vi "Test Prepare Path Returns Default if Empty.vi"(11 "Test Case In":refnum<class "Report Plugin Test.lvclass">) -> (0 "error out":errorcluster, 3 "Test Case Out":refnum<class "Report Plugin Test.lvclass">)   [LabVIEW 2020, in "Report Plugin Test.lvclass"]
uses:
  Report Plugin Test.lvclass
  C:/git/astemes-lunit/source/Framework/Report Plugin/Report Plugin.lvclass
  C:/Program Files (x86)/National Instruments/LabVIEW 2020/vi.lib/Astemes/LUnit/Test Case.lvclass
  <vilib>/Astemes/LUnit/Test Case.lvclass/Test Case.ctl
  <vilib>/Astemes/LUnit/Core/LUnit Test Case/Private/Append Fail Result.vi
  <vilib>/Astemes/LUnit/Core/LUnit Test Case/Private/Append Pass Result.vi
  <vilib>/Astemes/LUnit/Core/LUnit Test Case/Private/Run In UI.vi
  <vilib>/Utility/error.llb/Clear Errors.vi
  source/Framework/Report Plugin/Report Plugin.lvclass
  <vilib>/Astemes/LUnit/Test Case.lvclass
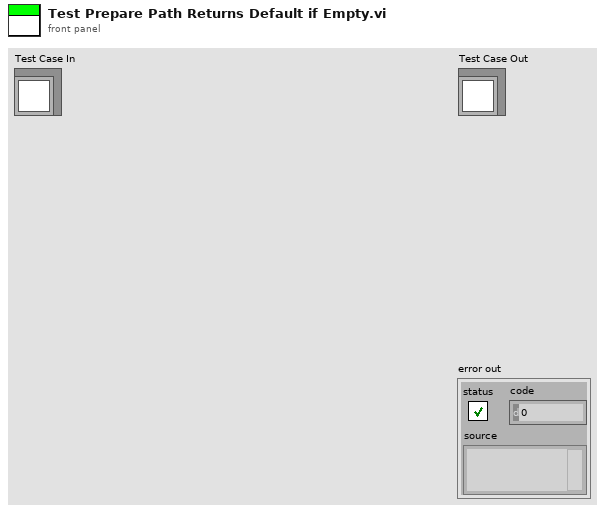
[diagram p1: front panel]
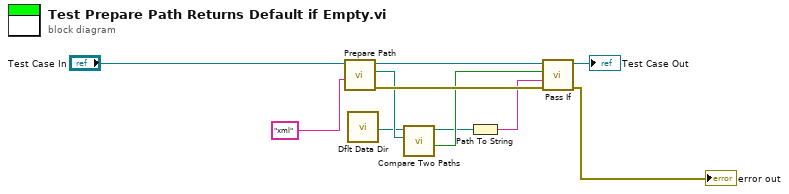
[diagram p0: block diagram]
diagram:
  n1 = call "Prepare Path.vi"("Extenssion"="xml", "Plugin In"="Test Case In") -> ("error out"=w7:errorcluster, "Modified Path"=w5:path, "Plugin Out"=w8:refnum<class "Report Plugin Test.lvclass">)  [unwired: 7 in]
  n2 = call <vilib>:"Dflt Data Dir.vi"() -> ("App:Default Data Directory"=w4:path)
  n3 = call <vilib>:"Compare Two Paths.vi"("Path 2"=w5, "Path 1"=w4) -> ("Path 2 Relative to Path 1?"=w3:bool, "Relative Path from 1 to 2"=w2:path)  [unwired: 6 in, 2 out]
  n4 = Path To String(path=w2) -> (string=w1:string)
  n5 = call <vilib>:"Pass If.vi"("error in (no error)"=w7, "Message"=w1, "Pass?"=w3, "LUnit Test Case In"=w8) -> ("error out"=→"error out":errorcluster, "LUnit Test Case Out"=→"Test Case Out":refnum<class "Report Plugin Test.lvclass">)  [unwired: 6 in]
